vi "HEWH GEA3_StationB.vi"(8 "error in":errorcluster, 11 "Message Queues out":T1) -> (0 "error out":errorcluster)   [LabVIEW 2023]
uses:
  Tenney/support/Message Queue/All Message Queues.ctl
  Tenney/support/Message Queue/Message Cluster.ctl
  Type Definitions/HEWH GEA3 Data.ctl
  Drivers/GEA3 Toolkit/LabVIEW GEA3 Rev2 API Toolkit LV2016/Water Heating Specific/Type Definitions/GEA3 HEWH ERD Data.ctl
  Drivers/GEA3 Toolkit/LabVIEW GEA3 Rev2 API Toolkit LV2016/Water Heating Specific/Type Definitions/GEA3 HEWH Mixing Valve.ctl
  Drivers/GEA3 Toolkit/LabVIEW GEA3 Rev2 API Toolkit LV2016/type defs/ERD Write Data In.ctl
  Drivers/GEA3 Toolkit/LabVIEW GEA3 Rev2 API Toolkit LV2016/type defs/Data Type.ctl
  Utility/Save File/File Setup (Public)/Type Definition/Save File HEWH Heating Control Mode.ctl
  Drivers/GEA3 Toolkit/LabVIEW GEA3 Rev2 API Toolkit LV2016/Water Heating Specific/Type Definitions/GEA3 HEWH Personality.ctl
  FVIR and LDO/support/Message Queue/Enqueue Message (Single).vi
  FVIR and LDO/support/Message Queue/Message Queue.lvlib
  Drivers/GEA3 Toolkit/LabVIEW GEA3 Rev2 API Toolkit LV2016/library/GEA2_Toolkit.lvlib
  Utility/Save File/File Setup.lvlib
  Tenney/support/Message Queue/Tenney Message Queue.lvlib
panel:
  out "Loop Count":i32
  in  "Pink Bean Board Index":i32
  out "Pink Bean Board ID":string
  in  "Debug":bool
  out "Debug":string[](array[string])
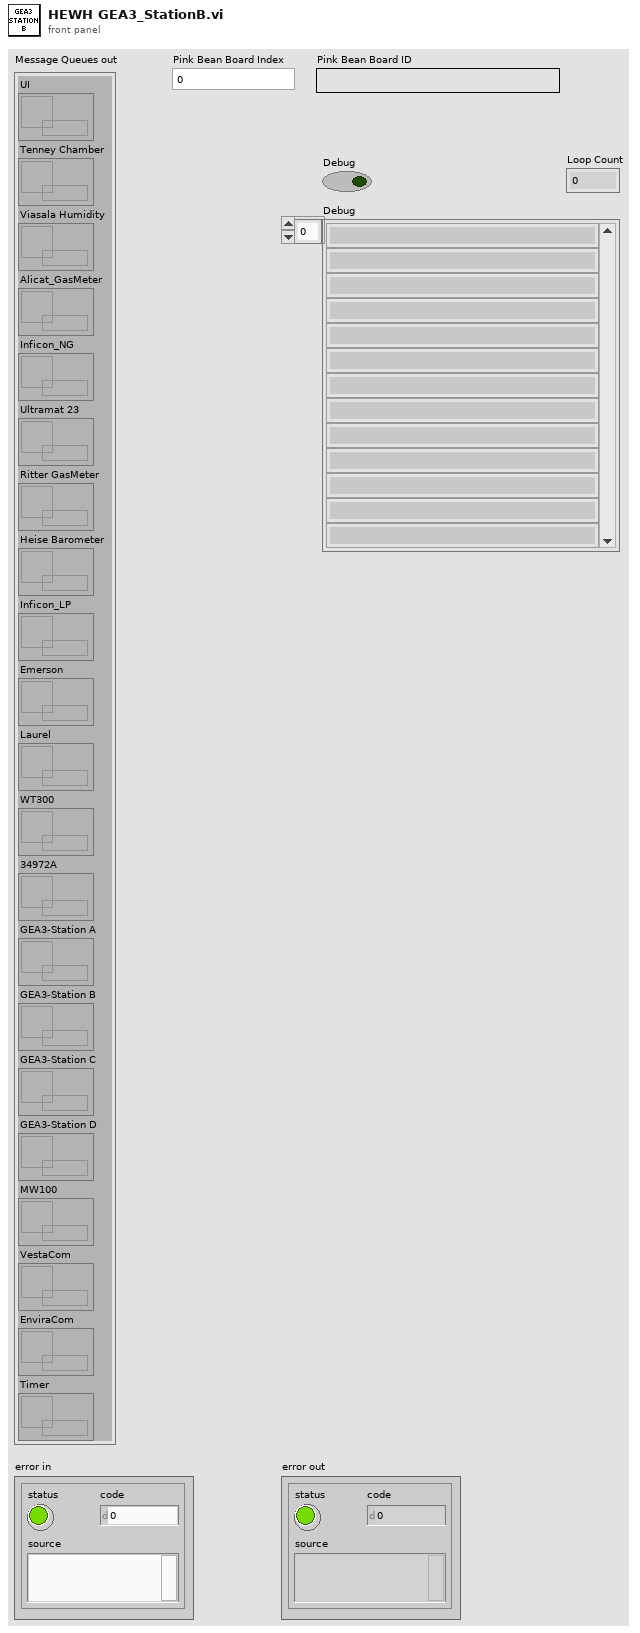
[diagram p1: front panel]
types:
  T1 = typedef "Tenney Message Queue.lvlib/All Message Queues.ctl" = cluster{"UI":refnum<queue>, "Tenney Chamber":refnum<queue>, "Viasala Humidity":refnum<queue>, "Alicat_GasMeter":refnum<queue>, "Inficon_NG":refnum<queue>, "Ultramat 23":refnum<queue>, "Ritter GasMeter":refnum<queue>, "Heise Barometer":refnum<queue>, "Inficon_LP":refnum<queue>, "Emerson":refnum<queue>, "Laurel":refnum<queue>, "WT300":refnum<queue>, "34972A":refnum<queue>, "GEA3-Station A":refnum<queue>, "GEA3-Station B":refnum<queue>, "GEA3-Station C":refnum<queue>, "GEA3-Station D":refnum<queue>, "MW100":refnum<queue>, "VestaCom":refnum<queue>, "EnviraCom":refnum<queue>, "Timer":refnum<queue>}
  T2 = typedef "HEWH GEA3 Data.ctl" = cluster{"ERD Data Input":T3, "ERD Data":string[][]}
  T3 = typedef "GEA3 HEWH ERD Data.ctl" = cluster{"Mixing Valve":T4, "Standard ERDs":cluster{"User UI Mode (0X4020)":string, "User Setpoint (0x4024)":u16, "Compressor (0x4068)":bool, "Lower Element (0x4068)":bool, "Upper Element (0x4068)":bool, "Fan (0x4068)":bool, "T1 Temp Lower Tank (°F) - (0x405F)":dbl, "T2 Temp Upper Tank (°F) - (0x4060)":dbl, "Line Voltage (0x4066)":u16, "MeasuredCurrent (0x4065)":dbl, "Tank Setpoint (°F) - (0x4026)":u16, "Depletion - (0x40CB)":u16, "Personality - (0x0035)":u16}, "Heat Pump":cluster{"EEV Position - (0X4067)":u16, "T3A TEMP EVAP IN (°F) - (0x4061)":dbl, "T3B TEMP EVAP OUT (°F) -(0x4062)":dbl, "T4 TEMP COMP DISCHARGE (°F) - (0x4063)":dbl, "T5 TEMP AMBIENT (°F)- (0x4064)":dbl, "Condensate Sensor - (0x40BC)":u16, "Fan (RPM) - (0xF073)":u16, "PWM (%) - (0xF056)":u16, "Compressor Speed (RPM) - (0xF093)":u16, "Compressor Target (RPM) - (0xF081)":u16, "Compressor Power (W) - (0xF092)":u16, "CPU Temperature (°F) - (0x40BA)":dbl, "Board Temperature (°F) - (0x40BB)":dbl}, "Inverter":cluster{"Inverter IGBT Temp (°C) - (0xF280)":dbl, "Inverter Chip Temp (°C) - (0xF284)":dbl}}
  T4 = typedef "GEA3 HEWH Mixing Valve.ctl" = cluster{"T7 Temp (°F) - (0x40B9)":dbl, "MixValveAbsoluteStepPosition - (0x400B)":i16, "Flow State - (0X4069)":u8, "T6 Temp (°F) - (0x406E)":dbl}
  T5 = typedef "GEA2_Toolkit.lvlib/ERD Write Data In.ctl" = cluster{"ERD Number":u16, "Data Type":T6, "Data":string}
  T6 = typedef "GEA2_Toolkit.lvlib/Data Type.ctl" = enum16{"string", "boolean", "uint8_t", "uint16_t", "uint32_t", "uint64_t", "int8_t", "int16_t", "int32_t", "int64_t"}
  T7 = typedef "File Setup.lvlib/Save File HEWH Heating Control Mode.ctl" = string
  T8 = typedef "GEA3 HEWH Personality.ctl" = string
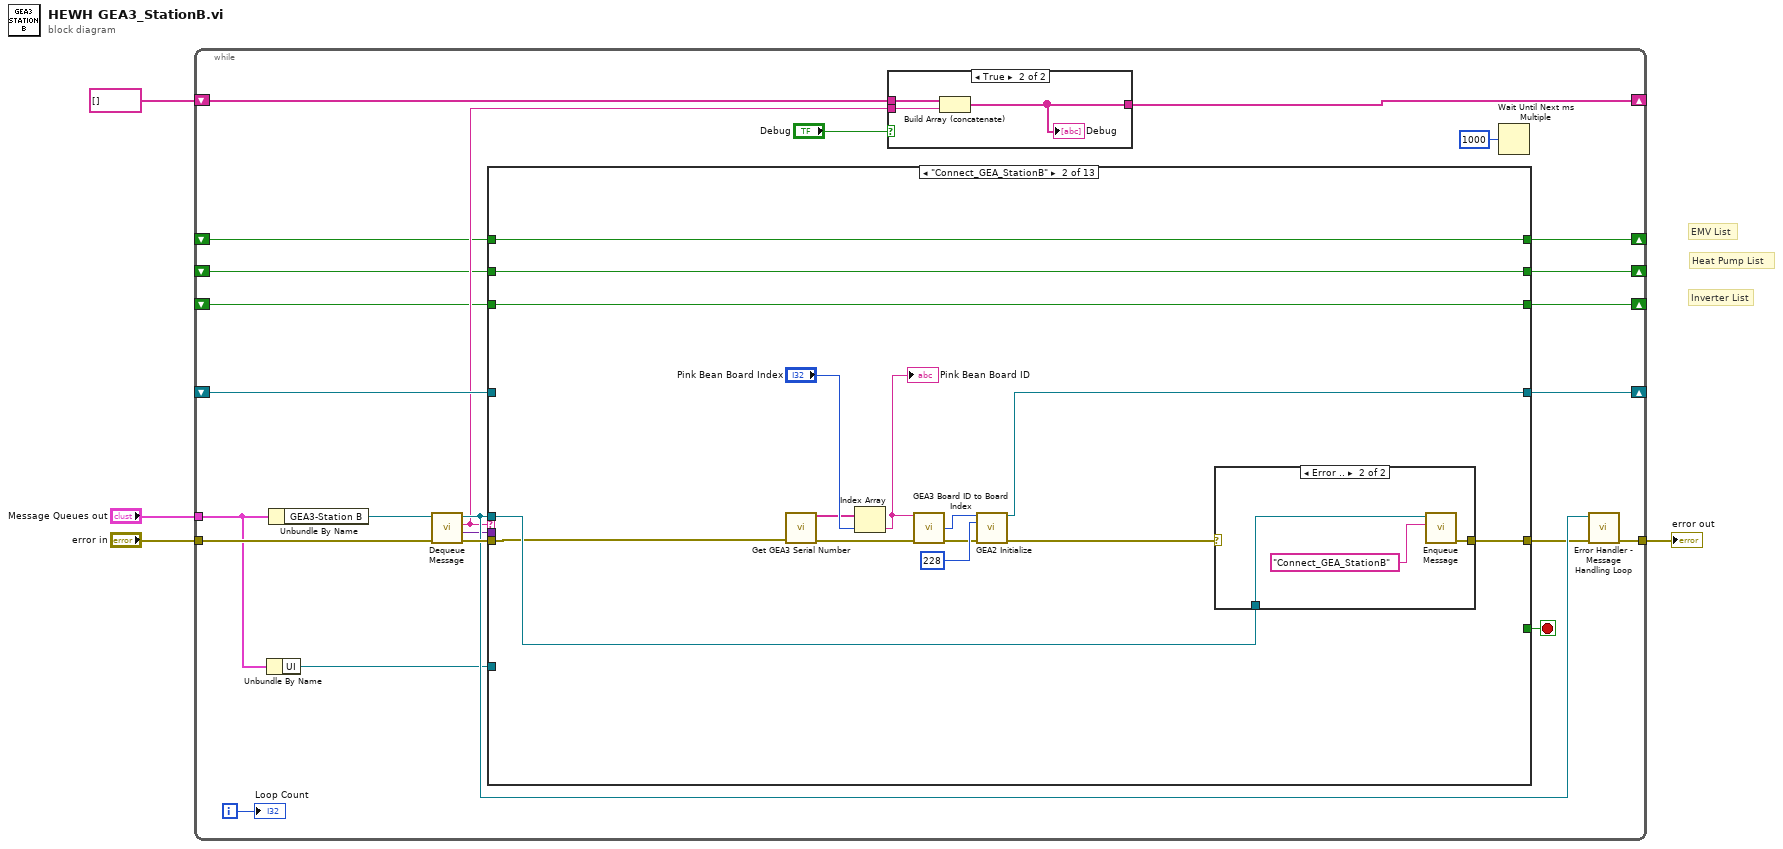
[diagram p0: block diagram]
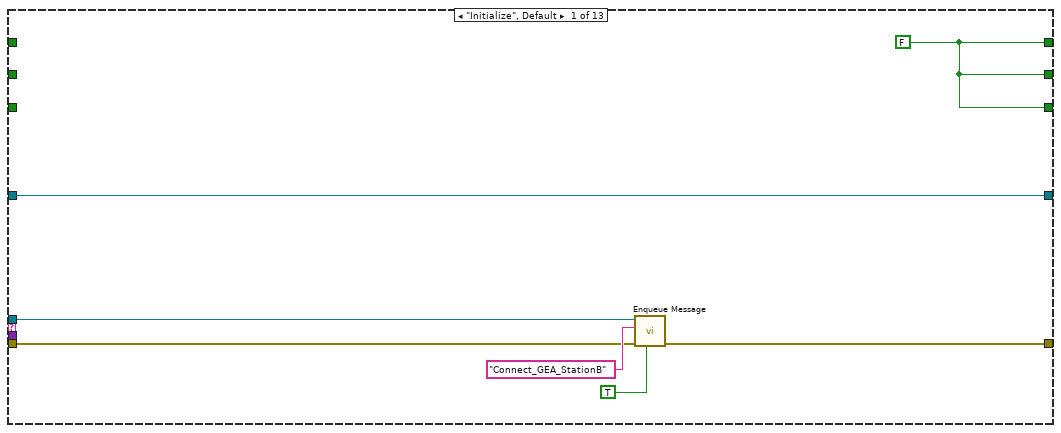
[diagram p3: hidden frame]
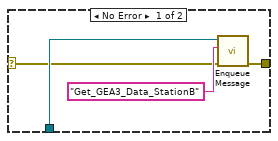
[diagram p4: hidden frame]
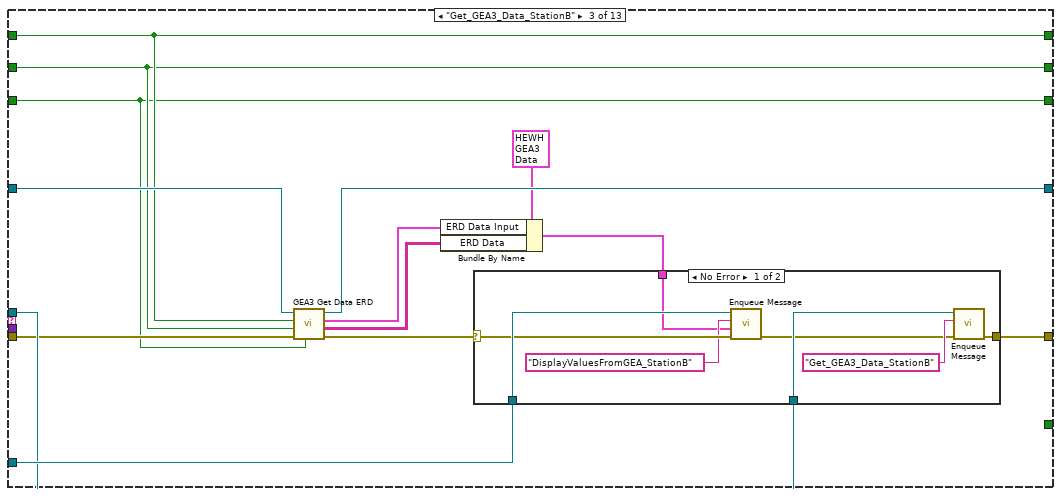
[diagram p5: hidden frame]
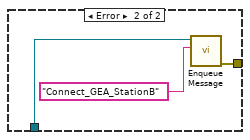
[diagram p6: hidden frame]
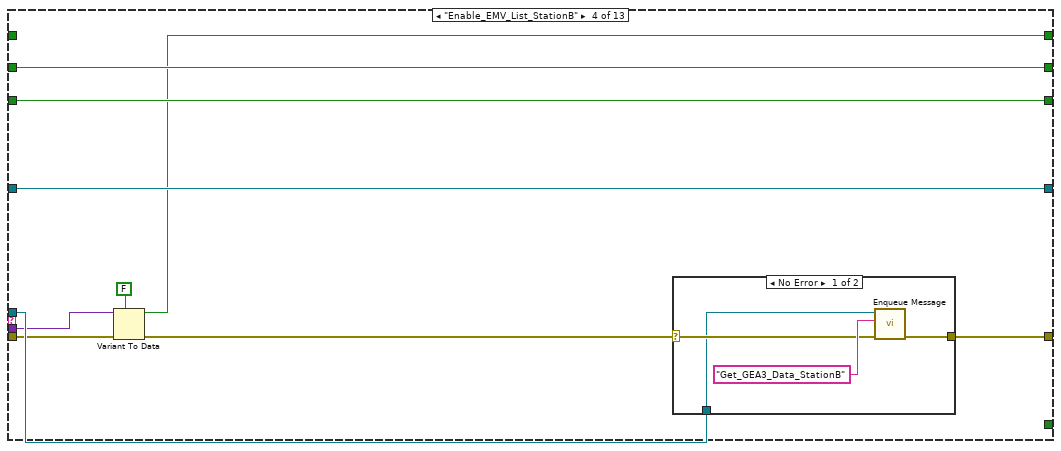
[diagram p7: hidden frame]
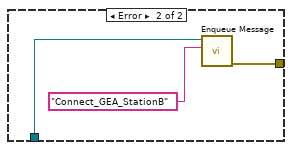
[diagram p8: hidden frame]
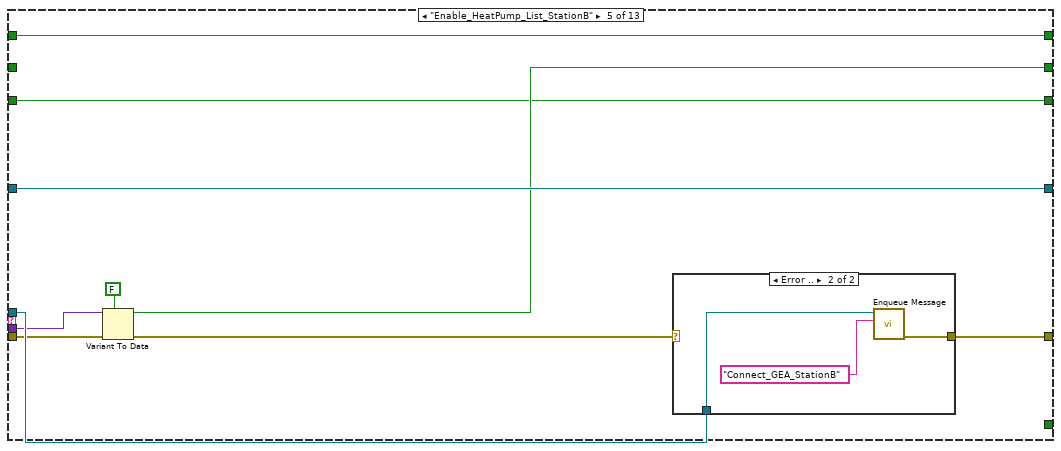
[diagram p9: hidden frame]
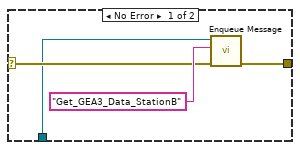
[diagram p10: hidden frame]
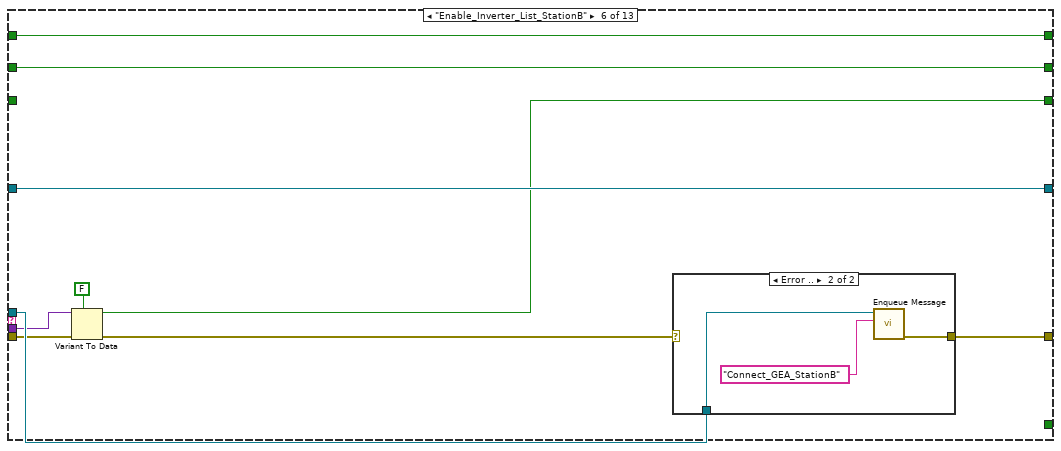
[diagram p11: hidden frame]
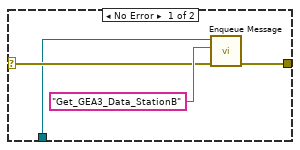
[diagram p12: hidden frame]
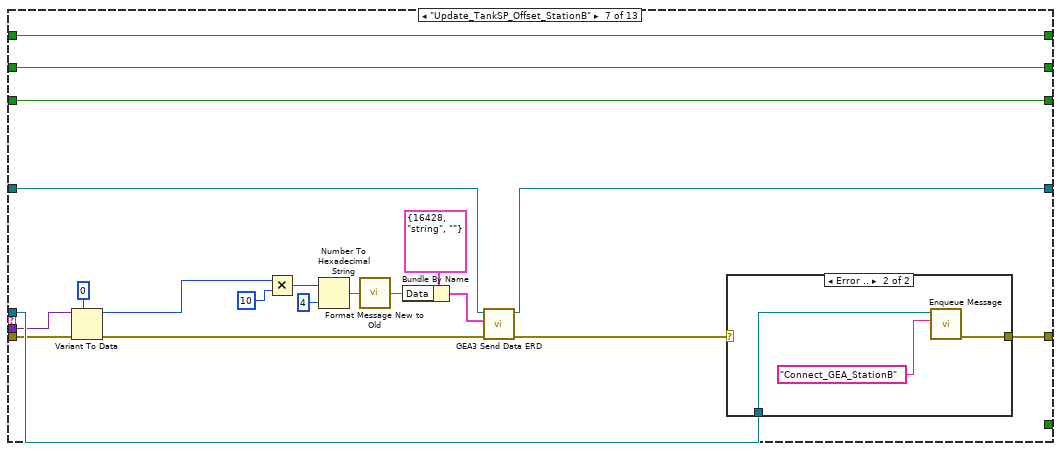
[diagram p13: hidden frame]
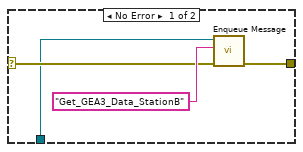
[diagram p14: hidden frame]
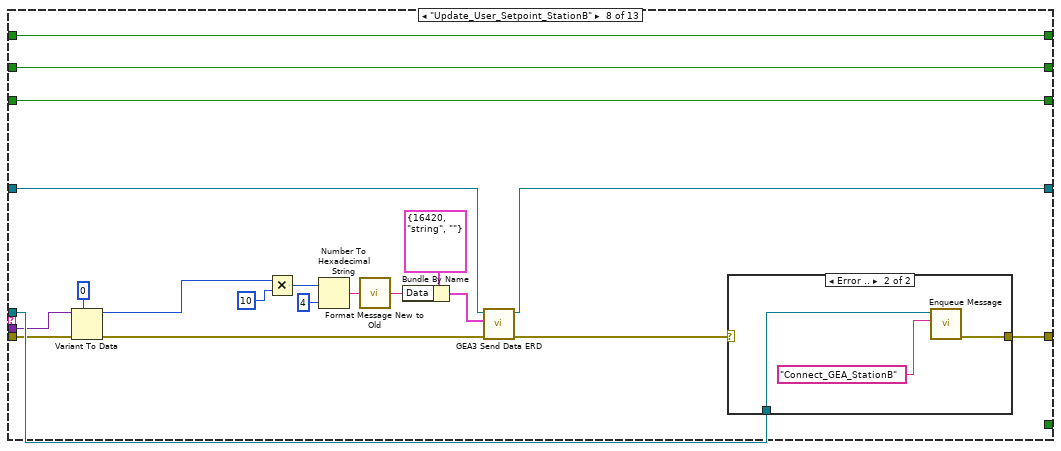
[diagram p15: hidden frame]
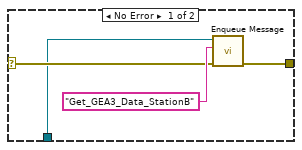
[diagram p16: hidden frame]
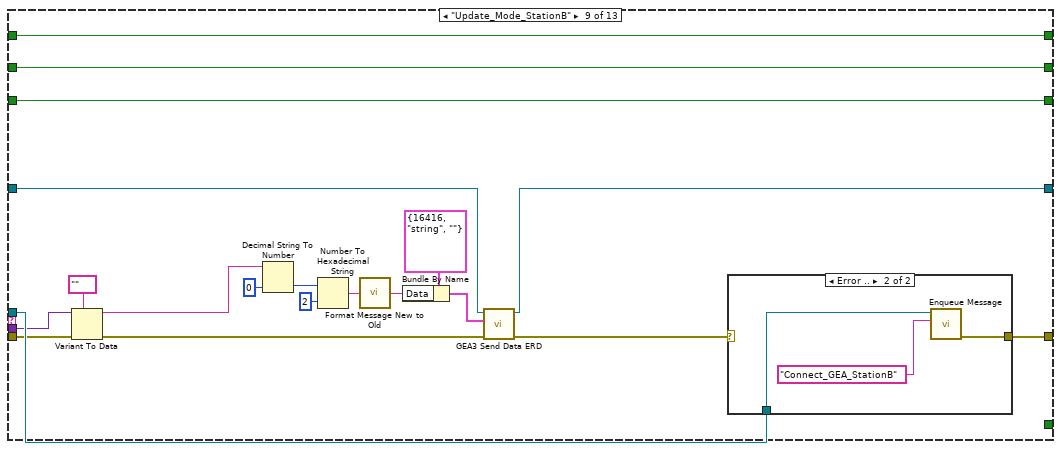
[diagram p17: hidden frame]
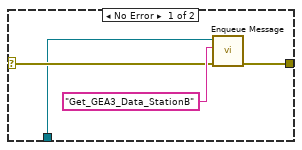
[diagram p18: hidden frame]
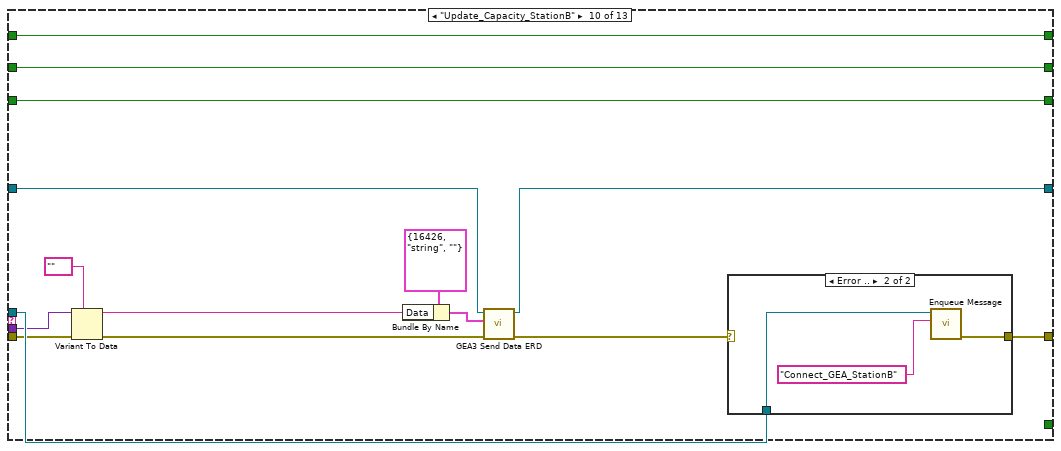
[diagram p19: hidden frame]
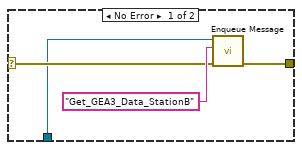
[diagram p20: hidden frame]
diagram:
  # "Inverter List"
  # "Heat Pump List"
  # "EMV List"
  n1 = while {
    tunnel: "Message Queues out" -> [w18]
    tunnel: "error in" -> [w27]
    tunnel: [w23] -> w3
    shift-right: [w21] -> _
    shift-left: _ -> [w20]
    shift-right: [w14] -> _
    shift-left: string[] [] -> [w15]
    shift-right: [w12] -> _
    shift-left: _ -> [w9]
    shift-right: [w11] -> _
    shift-left: _ -> [w8]
    shift-right: [w10] -> _
    shift-left: _ -> [w7]
    i -> [w5]
    stop <- w25 stop-if-true
    n2 = Unbundle By Name(w18) -> ("UI"=w17:refnum<queue>)
    n3 = Unbundle By Name(w18) -> ("GEA3-Station B"=w28:refnum<queue>)
    n4 = call "Dequeue Message.vi"("error in (no error)"=w27, "Message Queue"=w28) -> ("error out"=w26:errorcluster, "Message Data"=w6:variant, "Message"=w16:string, "dup Message Queue"=w24:refnum<queue>)  [unwired: 6 in]
    n5 = case shown="\"Connect_GEA_StationB\"" w16 {
      tunnel: w26 -> [w37 w45 w72 w91 w109 w126 w155 w182 w209 w231 w255 w266 w294]
      tunnel: [w36 w54 w74 w96 w113 w130 w157 w184 w211 w233 w257 w280 w289] -> w22
      tunnel: [_ _ _ _ _ _ _ _ _ _ _ _ TRUE] -> w25
      tunnel: w24 -> [w35 w53 w73 w95 w112 w129 w156 w183 w210 w232 w256 w279 w295]
      tunnel: [w39 w43 w70 w94 w111 w128 w142 w169 w202 w224 w249 w274 w288] -> w21
      tunnel: w20 -> [w39 _ w69 w94 w111 w128 w143 w170 w203 w225 w250 w275 w288]
      tunnel: w17 -> [_ _ w75 _ _ _ _ _ _ _ _ _ _]
      tunnel: [w33 w42 w68 w87 w105 w122 w153 w180 w207 w229 w253 w278 w293] -> w12
      tunnel: [w33 w41 w67 w93 w106 w121 w152 w179 w206 w228 w252 w277 w292] -> w11
      tunnel: [w33 w40 w66 w92 w104 w123 w138 w165 w199 w221 w246 w272 w291] -> w10
      tunnel: w9 -> [_ w42 w68 _ w105 w122 w153 w180 w207 w229 w253 w278 w293]
      tunnel: w8 -> [_ w41 w67 w93 _ w121 w152 w179 w206 w228 w252 w277 w292]
      tunnel: w7 -> [_ w40 w66 w92 w104 _ w138 w165 w199 w221 w246 w272 w291]
      tunnel: w6 -> [_ _ _ w89 w107 w124 w154 w181 w208 w230 w254 _ _]
      frame "Initialize", Default {
        w33 = FALSE
        n6 = call-poly "Enqueue Message.vi"("Priority Message? (F)"=TRUE, "error in (no error)"=w37, "Message"="Connect_GEA_StationB", "Message Queue"=w35) -> ("error out"=w36:errorcluster)  [unwired: 6 in, 1 out]
      }
      frame "Connect_GEA_StationB" {
        n7 = call "Get GEA3 Serial Number.vi"("Error In"=w45) -> ("GEA3 Serial Numbers"=w49:string[], "Error Out"=w48:errorcluster)  [unwired: 13 in]
        n8 = Index Array(array=w49, index="Pink Bean Board Index") -> (element=w50:string)
        "Pink Bean Board ID" <- w50
        n9 = call "GEA3 Board ID to Board Index.vi"("GEA3 Serial Number"=w50, "Error In"=w48) -> ("Board Index"=w47:i32, "Error Out"=w46:errorcluster)  [unwired: 9 in, 3 out]
        n10 = call "GEA2 Initialize.vi"("Board Index"=w47, "Source Address"=u8 228, "error in"=w46) -> ("GEA2 Reference Out"=w43:refnum<k24>, "error out"=w44:errorcluster)  [unwired: 10 in, 1 out]
        n11 = case shown="Error .." w44 {
          selector: w44 -> [w55 _]
          tunnel: [w57 w60] -> w54
          tunnel: w53 -> [w56 w59]
          frame No Error {
            n12 = call-poly "Enqueue Message.vi"("error in (no error)"=w55, "Message"="Get_GEA3_Data_StationB", "Message Queue"=w56) -> ("error out"=w57:errorcluster)  [unwired: 7 in, 1 out]
          }
          frame Error {
            n13 = call-poly "Enqueue Message.vi"("Message"="Connect_GEA_StationB", "Message Queue"=w59) -> ("error out"=w60:errorcluster)  [unwired: 8 in, 1 out]
          }
        }
      }
      frame "Get_GEA3_Data_StationB" {
        n14 = call "GEA3 Get Data ERD.vi"("Enable Inverter ERD List"=w66, "error in (no error)"=w72, "Enable Heat Pump List"=w67, "Enable EMV List"=w68, ".NET Refnum in"=w69) -> ("error out"=w71:errorcluster, "ERD Data"=w64:string[][], "ERD Data Input"=w63:T3, ".NET Refnum out"=w70:refnum<k24>)  [unwired: 3 in]
        n15 = Bundle By Name(cluster=T2 {"ERD Data Input"={"Mixing Valve"={"T7 Temp (°F) - (0x40B9)"=0.0, "MixValveAbsoluteStepPosition - (0x400B)"=0, "Flow State - (0X4069)"=0, "T6 Temp (°F) - (0x406E)"=0.0}, "Standard ERDs"={"User UI Mode (0X4020)"="", "User Setpoint (0x4024)"=0, "Compressor (0x4068)"=FALSE, "Lower Element (0x4068)"=FALSE, "Upper Element (0x4068)"=FALSE, "Fan (0x4068)"=FALSE, "T1 Temp Lower Tank (°F) - (0x405F)"=0.0, "T2 Temp Upper Tank (°F) - (0x4060)"=0.0, "Line Voltage (0x4066)"=0, "MeasuredCurrent (0x4065)"=0.0, "Tank Setpoint (°F) - (0x4026)"=0, "Depletion - (0x40CB)"=0, "Personality - (0x0035)"=0}, "Heat Pump"={"EEV Position - (0X4067)"=0, "T3A TEMP EVAP IN (°F) - (0x4061)"=0.0, "T3B TEMP EVAP OUT (°F) -(0x4062)"=0.0, "T4 TEMP COMP DISCHARGE (°F) - (0x4063)"=0.0, "T5 TEMP AMBIENT (°F)- (0x4064)"=0.0, "Condensate Sensor - (0x40BC)"=0, "Fan (RPM) - (0xF073)"=0, "PWM (%) - (0xF056)"=0, "Compressor Speed (RPM) - (0xF093)"=0, "Compressor Target (RPM) - (0xF081)"=0, "Compressor Power (W) - (0xF092)"=0, "CPU Temperature (°F) - (0x40BA)"=0.0, "Board Temperature (°F) - (0x40BB)"=0.0}, "Inverter"={"Inverter IGBT Temp (°C) - (0xF280)"=0.0, "Inverter Chip Temp (°C) - (0xF284)"=0.0}}, "ERD Data"=[]} ("GEA3 Data"), "ERD Data Input"=w63, "ERD Data"=w64) -> (w62:T2)
        n16 = case shown="No Error" w71 {
          selector: w71 -> [w78 _]
          tunnel: w75 -> [w83 _]
          tunnel: [w82 w85] -> w74
          tunnel: w73 -> [w81 w84]
          tunnel: w62 -> [w76 _]
          frame No Error {
            n17 = call-poly "Enqueue Message.vi"("error in (no error)"=w78, "Message Data"=w76, "Message"="DisplayValuesFromGEA_StationB", "Message Queue"=w83) -> ("error out"=w79:errorcluster)  [unwired: 6 in, 1 out]
            n18 = call-poly "Enqueue Message.vi"("error in (no error)"=w79, "Message"="Get_GEA3_Data_StationB", "Message Queue"=w81) -> ("error out"=w82:errorcluster)  [unwired: 7 in, 1 out]
          }
          frame Error {
            n19 = call-poly "Enqueue Message.vi"("Message"="Connect_GEA_StationB", "Message Queue"=w84) -> ("error out"=w85:errorcluster)  [unwired: 8 in, 1 out]
          }
        }
      }
      frame "Enable_EMV_List_StationB" {
        n20 = Variant To Data(error in=w91, type=FALSE, Variant=w89) -> (data=w87:bool, error out=w90:errorcluster)
        n21 = case shown="No Error" w90 {
          selector: w90 -> [w99 _]
          tunnel: [w98 w102] -> w96
          tunnel: w95 -> [w97 w101]
          frame No Error {
            n22 = call-poly "Enqueue Message.vi"("error in (no error)"=w99, "Message"="Get_GEA3_Data_StationB", "Message Queue"=w97) -> ("error out"=w98:errorcluster)  [unwired: 7 in, 1 out]
          }
          frame Error {
            n23 = call-poly "Enqueue Message.vi"("Message"="Connect_GEA_StationB", "Message Queue"=w101) -> ("error out"=w102:errorcluster)  [unwired: 8 in, 1 out]
          }
        }
      }
      frame "Enable_HeatPump_List_StationB" {
        n24 = Variant To Data(error in=w109, type=FALSE, Variant=w107) -> (data=w106:bool, error out=w108:errorcluster)
        n25 = case shown="Error .." w108 {
          selector: w108 -> [w116 _]
          tunnel: [w115 w119] -> w113
          tunnel: w112 -> [w114 w118]
          frame No Error {
            n26 = call-poly "Enqueue Message.vi"("error in (no error)"=w116, "Message"="Get_GEA3_Data_StationB", "Message Queue"=w114) -> ("error out"=w115:errorcluster)  [unwired: 7 in, 1 out]
          }
          frame Error {
            n27 = call-poly "Enqueue Message.vi"("Message"="Connect_GEA_StationB", "Message Queue"=w118) -> ("error out"=w119:errorcluster)  [unwired: 8 in, 1 out]
          }
        }
      }
      frame "Enable_Inverter_List_StationB" {
        n28 = Variant To Data(error in=w126, type=FALSE, Variant=w124) -> (data=w123:bool, error out=w125:errorcluster)
        n29 = case shown="Error .." w125 {
          selector: w125 -> [w133 _]
          tunnel: [w132 w136] -> w130
          tunnel: w129 -> [w131 w135]
          frame No Error {
            n30 = call-poly "Enqueue Message.vi"("error in (no error)"=w133, "Message"="Get_GEA3_Data_StationB", "Message Queue"=w131) -> ("error out"=w132:errorcluster)  [unwired: 7 in, 1 out]
          }
          frame Error {
            n31 = call-poly "Enqueue Message.vi"("Message"="Connect_GEA_StationB", "Message Queue"=w135) -> ("error out"=w136:errorcluster)  [unwired: 8 in, 1 out]
          }
        }
      }
      frame "Update_TankSP_Offset_StationB" {
        n32 = Variant To Data(error in=w155, type=i16 0, Variant=w154) -> (data=w139:i16, error out=w141:errorcluster)
        n33 = Multiply(x=w139, y=i16 10) -> (x*y=w150:i16)
        n34 = Number To Hexadecimal String(1:i16 4 ("width (-)"), 2:w150) -> (0:w148:string)
        n35 = call "Format Message New to Old.vi"("Raw Message In"=w148) -> ("Conv Message Out"=w145:string)  [unwired: 14 in]
        n36 = Bundle By Name(cluster=T5 {"ERD Number"=16428, "Data Type"=enum."string", "Data"=""} ("ERD Write Data In"), "Data"=w145) -> (w144:T5)
        n37 = call "GEA3 Send Data ERD.vi"("error in (no error)"=w141, "ERD Write Data In"=w144, ".NET Refnum in"=w143) -> ("error out"=w140:errorcluster, "GEA2 Reference Out"=w142:refnum<k24>)  [unwired: 5 in, 2 out]
        n38 = case shown="Error .." w140 {
          selector: w140 -> [w160 _]
          tunnel: [w159 w163] -> w157
          tunnel: w156 -> [w158 w162]
          frame No Error {
            n39 = call-poly "Enqueue Message.vi"("error in (no error)"=w160, "Message"="Get_GEA3_Data_StationB", "Message Queue"=w158) -> ("error out"=w159:errorcluster)  [unwired: 7 in, 1 out]
          }
          frame Error {
            n40 = call-poly "Enqueue Message.vi"("Message"="Connect_GEA_StationB", "Message Queue"=w162) -> ("error out"=w163:errorcluster)  [unwired: 8 in, 1 out]
          }
        }
      }
      frame "Update_User_Setpoint_StationB" {
        n41 = Variant To Data(error in=w182, type=i16 0, Variant=w181) -> (data=w166:i16, error out=w168:errorcluster)
        n42 = Multiply(x=w166, y=i16 10) -> (x*y=w177:i16)
        n43 = Number To Hexadecimal String(1:i16 4 ("width (-)"), 2:w177) -> (0:w175:string)
        n44 = call "Format Message New to Old.vi"("Raw Message In"=w175) -> ("Conv Message Out"=w172:string)  [unwired: 14 in]
        n45 = Bundle By Name(cluster=T5 {"ERD Number"=16420, "Data Type"=enum."string", "Data"=""} ("ERD Write Data In"), "Data"=w172) -> (w171:T5)
        n46 = call "GEA3 Send Data ERD.vi"("error in (no error)"=w168, "ERD Write Data In"=w171, ".NET Refnum in"=w170) -> ("error out"=w167:errorcluster, "GEA2 Reference Out"=w169:refnum<k24>)  [unwired: 5 in, 2 out]
        n47 = case shown="Error .." w167 {
          selector: w167 -> [w187 _]
          tunnel: [w186 w190] -> w184
          tunnel: w183 -> [w185 w189]
          frame No Error {
            n48 = call-poly "Enqueue Message.vi"("error in (no error)"=w187, "Message"="Get_GEA3_Data_StationB", "Message Queue"=w185) -> ("error out"=w186:errorcluster)  [unwired: 7 in, 1 out]
          }
          frame Error {
            n49 = call-poly "Enqueue Message.vi"("Message"="Connect_GEA_StationB", "Message Queue"=w189) -> ("error out"=w190:errorcluster)  [unwired: 8 in, 1 out]
          }
        }
      }
      frame "Update_Mode_StationB" {
        n50 = Variant To Data(error in=w209, type=T7 "" ("Heating Mode."), Variant=w208) -> (data=w193:T7, error out=w201:errorcluster)
        n51 = Decimal String To Number(string=w193, default (0L)=u16 0 ("default (0 I32)")) -> (number=w197:u16)  [unwired: 1 in, 1 out]
        n52 = Number To Hexadecimal String(1:i16 2 ("width (-)"), 2:w197) -> (0:w198:string)
        n53 = call "Format Message New to Old.vi"("Raw Message In"=w198) -> ("Conv Message Out"=w192:string)  [unwired: 14 in]
        n54 = Bundle By Name(cluster=T5 {"ERD Number"=16416, "Data Type"=enum."string", "Data"=""} ("ERD Write Data In"), "Data"=w192) -> (w204:T5)
        n55 = call "GEA3 Send Data ERD.vi"("error in (no error)"=w201, "ERD Write Data In"=w204, ".NET Refnum in"=w203) -> ("error out"=w200:errorcluster, "GEA2 Reference Out"=w202:refnum<k24>)  [unwired: 5 in, 2 out]
        n56 = case shown="Error .." w200 {
          selector: w200 -> [w214 _]
          tunnel: [w213 w217] -> w211
          tunnel: w210 -> [w212 w216]
          frame No Error {
            n57 = call-poly "Enqueue Message.vi"("error in (no error)"=w214, "Message"="Get_GEA3_Data_StationB", "Message Queue"=w212) -> ("error out"=w213:errorcluster)  [unwired: 7 in, 1 out]
          }
          frame Error {
            n58 = call-poly "Enqueue Message.vi"("Message"="Connect_GEA_StationB", "Message Queue"=w216) -> ("error out"=w217:errorcluster)  [unwired: 8 in, 1 out]
          }
        }
      }
      frame "Update_Capacity_StationB" {
        n59 = Variant To Data(error in=w231, type="" ("Capacity Setting"), Variant=w230) -> (data=w219:string, error out=w223:errorcluster)
        n60 = Bundle By Name(cluster=T5 {"ERD Number"=16426, "Data Type"=enum."string", "Data"=""} ("ERD Write Data In"), "Data"=w219) -> (w226:T5)
        n61 = call "GEA3 Send Data ERD.vi"("error in (no error)"=w223, "ERD Write Data In"=w226, ".NET Refnum in"=w225) -> ("error out"=w222:errorcluster, "GEA2 Reference Out"=w224:refnum<k24>)  [unwired: 5 in, 2 out]
        n62 = case shown="Error .." w222 {
          selector: w222 -> [w236 _]
          tunnel: [w235 w239] -> w233
          tunnel: w232 -> [w234 w238]
          frame No Error {
            n63 = call-poly "Enqueue Message.vi"("error in (no error)"=w236, "Message"="Get_GEA3_Data_StationB", "Message Queue"=w234) -> ("error out"=w235:errorcluster)  [unwired: 7 in, 1 out]
          }
          frame Error {
            n64 = call-poly "Enqueue Message.vi"("Message"="Connect_GEA_StationB", "Message Queue"=w238) -> ("error out"=w239:errorcluster)  [unwired: 8 in, 1 out]
          }
        }
      }
      frame "Update_Personality_StationB" {
        n65 = Variant To Data(error in=w255, type=T8 "" ("Personality"), Variant=w254) -> (data=w243:T8, error out=w248:errorcluster)
        n66 = Bundle By Name(cluster=T5 {"ERD Number"=0, "Data Type"=enum."string", "Data"=""} ("ERD Write Data In"), "ERD Number"=u16 53, "Data Type"=Data_Type."string", "Data"=w243) -> (w251:T5)
        n67 = call "GEA3 Send Data ERD.vi"("error in (no error)"=w248, "ERD Write Data In"=w251, ".NET Refnum in"=w250) -> ("error out"=w247:errorcluster, "GEA2 Reference Out"=w249:refnum<k24>)  [unwired: 5 in, 2 out]
        n68 = case shown="Error .." w247 {
          selector: w247 -> [w260 _]
          tunnel: [w259 w263] -> w257
          tunnel: w256 -> [w258 w262]
          frame No Error {
            n69 = call-poly "Enqueue Message.vi"("error in (no error)"=w260, "Message"="Get_GEA3_Data_StationB", "Message Queue"=w258) -> ("error out"=w259:errorcluster)  [unwired: 7 in, 1 out]
          }
          frame Error {
            n70 = call-poly "Enqueue Message.vi"("Message"="Connect_GEA_StationB", "Message Queue"=w262) -> ("error out"=w263:errorcluster)  [unwired: 8 in, 1 out]
          }
        }
      }
      frame "Reset_Control_Counter_StationB" {
        n71 = Number To Hexadecimal String(1:i16 4 ("width (-)"), 2:0 ("number")) -> (0:w265:string)
        n72 = Bundle By Name(cluster=T5 {"ERD Number"=0, "Data Type"=enum."string", "Data"=""} ("ERD Write Data In"), "ERD Number"=u16 16576, "Data Type"=Data_Type."string", "Data"=w265) -> (w276:T5)
        n73 = call "GEA3 Send Data ERD.vi"("error in (no error)"=w266, "ERD Write Data In"=w276, ".NET Refnum in"=w275) -> ("error out"=w273:errorcluster, "GEA2 Reference Out"=w274:refnum<k24>)  [unwired: 5 in, 2 out]
        n74 = case shown="Error .." w273 {
          selector: w273 -> [w283 _]
          tunnel: [w282 w286] -> w280
          tunnel: w279 -> [w281 w285]
          frame No Error {
            n75 = call-poly "Enqueue Message.vi"("error in (no error)"=w283, "Message"="Get_GEA3_Data_StationB", "Message Queue"=w281) -> ("error out"=w282:errorcluster)  [unwired: 7 in, 1 out]
          }
          frame Error {
            n76 = call-poly "Enqueue Message.vi"("Message"="Connect_GEA_StationB", "Message Queue"=w285) -> ("error out"=w286:errorcluster)  [unwired: 8 in, 1 out]
          }
        }
      }
      frame "Exit" {
        n77 = Release Queue(queue=w295, error in (no error)=w294) -> (error out=w290:errorcluster)  [unwired: 1 in, 2 out]
        n78 = call "GEA2 Stop.vi"("GEA2 Reference In"=w288, "Error In"=w290) -> ("Error Out"=w289:errorcluster)  [unwired: 13 in]
      }
    }
    n79 = case shown="True" "Debug" {
      tunnel: w16 -> [_ w32]
      tunnel: w15 -> [w29 w31]
      tunnel: [w29 w30] -> w14
      frame False {
      }
      frame True {
        n80 = Build Array (concatenate)(w31, w32) -> (w30:string[])
        "Debug" <- w30
      }
    }
    n81 = Wait Until Next ms Multiple(millisecond multiple=u32 1000) -> ()  [unwired: 1 out]
    n82 = call "Error Handler - Message Handling Loop.vi"("error in (no error)"=w22, "Message Queue"=w24) -> ("dup error in"=w23:errorcluster)  [unwired: 8 in, 1 out]
    "Loop Count" <- w5
  }
  "error out" <- w3
